vi "Ordina nome colonne.vi"(10 "Array nomi":string[](array[string]), 11 "Array indici":string[](array[string])) -> (3 "Array nomi ordinati":string[](array[string]))   [LabVIEW 2019]
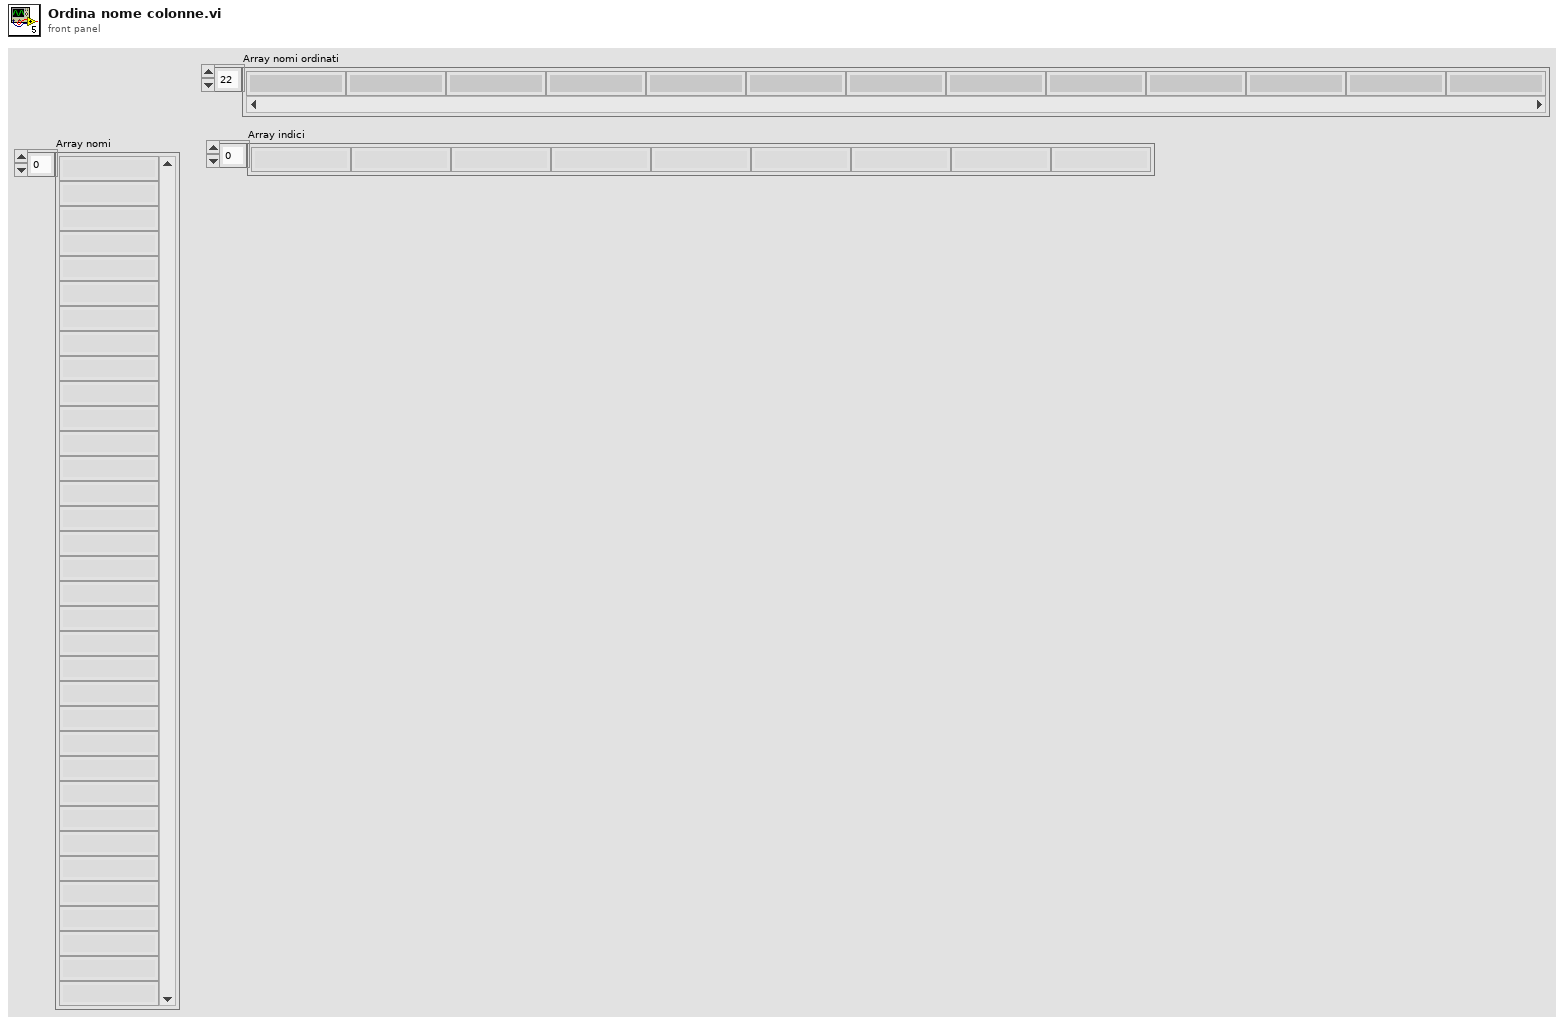
[diagram p1: front panel]
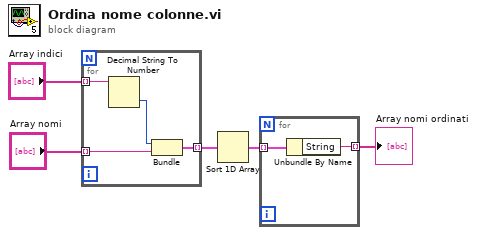
[diagram p0: block diagram]
diagram:
  n1 = for {
    tunnel: "Array indici" -> [w9] mode=indexing
    tunnel: [w7] -> w2 mode=indexing
    tunnel: "Array nomi" -> [w6] mode=indexing
    n2 = Decimal String To Number(string=w9) -> (number=w8:i32)  [unwired: 2 in, 1 out]
    n3 = Bundle(w8, "String"=w6) -> (w7:cluster{i32, "String":string})  [unwired: 1 in]
  }
  n4 = Sort 1D Array(array=w2) -> (sorted array=w4:cluster{i32, "String":string}[])
  n5 = for {
    tunnel: w4 -> [w11] mode=indexing
    tunnel: [w10] -> w5 mode=indexing
    n6 = Unbundle By Name(w11) -> ("String"=w10:string)
  }
  "Array nomi ordinati" <- w5
